vi "发送报文全局变量.vi"() -> ()   [LabVIEW 2016, in "环境动力监测库.lvlib" / "NMEA.lvlib"]
uses:
  NMEA.lvlib
panel:
  in  "接收命令":string
  in  "发送报文":string
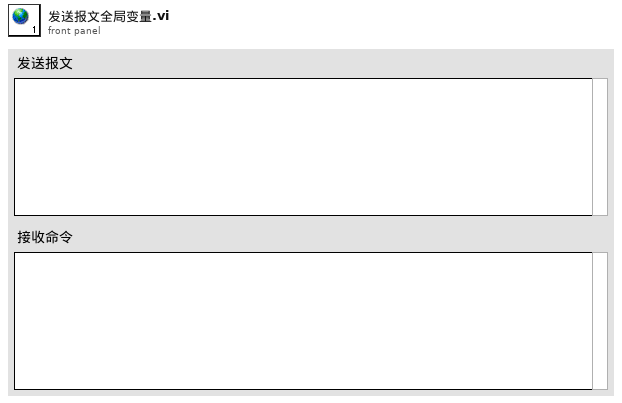
[diagram p1: front panel]
diagram:
